vi "FuncImg-Export full data.vi"() -> (0 "error out":errorcluster, 11 "Exported file path":path)   [LabVIEW 2017]
uses:
  <userlib>/_MGI/File/MGI Windows Folder Enum.ctl
  Experiment header interface/Typedefs/Header parameters cluster-Zstack.ctl
  Typedefs/Frame Size.ctl
  Global variables/gl_Functional Imaging-Global variables.vi
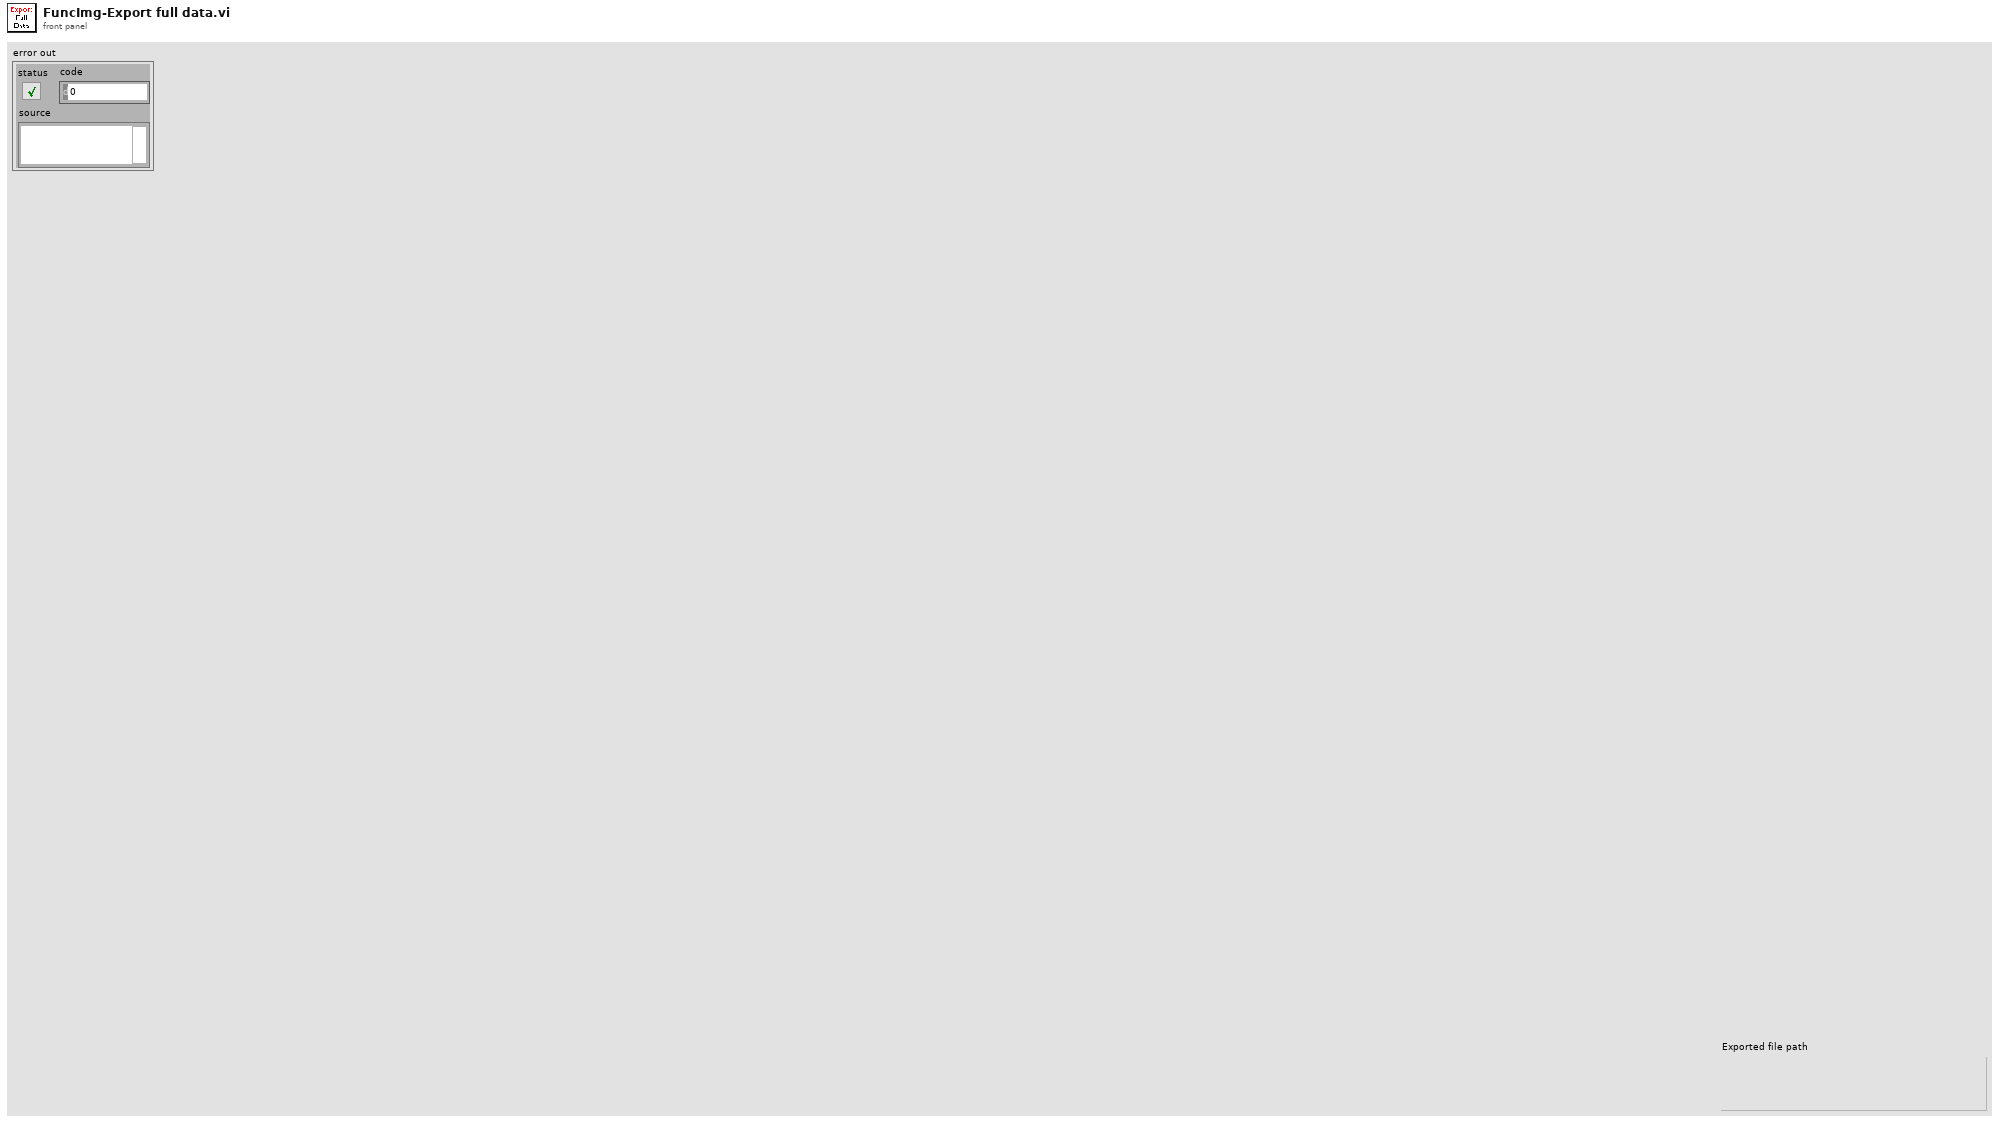
[diagram p1: front panel]
types:
  T1 = typedef "MGI Windows Folder Enum.ctl" = enum32{"Desktop", "Err<Internet>", "Programs", "Err<Controls>", "Err<Printers>", "Personal (MyDocuments)", "Favorites", "Startup", "Recent", "SendTo", "Err<RecycleBin>", "StartMenu", "Err<MyDocuments>", "MyMusic", "MyVideo", "Err<0x000F>", "DesktopDirectory", "Err<Drives>", "Err<Network>", "NetHood", "Fonts", "Templates", "CommonStartMenu", "CommonPrograms", "CommonStartup", "CommonDesktopDirectory", "AppData", "PrintHood", "LocalAppData", "Err<AltStartup>", "Err<CommonAltStartup>", "CommonFavorites", "InternetCache", "Cookies", "History", "CommonAppData", "Windows", "System", "ProgramFiles", "MyPictures", "Profile", "System32", "Err<0x002A>", "ProgramFilesCommon", "Err<0x002C>", "CommonTemplates", "CommonDocuments", "CommonAdminTools", "AdminTools"}
  T2 = typedef "Header parameters cluster-Zstack.ctl" = cluster{"Number of POI":u16, "Number of Miniscans":u16, "Number of Trials":u16, "Number of Cycles ":u16, "# Averaged Frames":u16, "Laser power (%)":u8, "Pockels":dbl, "Acquisition Length (sec)":dbl, "Fill time (us)":dbl, "DwellTime (us)":dbl, "Miniscan Dwell time per pixel (us)":dbl, "PMT 1":dbl, "PMT 2":dbl, "Back Apperture":dbl, "Zoom":dbl, "Number of Pixels in Miniscan":u16, "Frame Size":T3, "Field of View":dbl, "X centre":dbl, "Y centre":dbl, "AOL Z":dbl}
  T3 = typedef "Frame Size.ctl" = u16
  T4 = cluster{"Channel A?":bool, "Cycle length (us)":dbl, "[Pixels in ROI]":i32[], "Z-Stack Header data":T2, "[ROI Time (us)]":dbl[], "Path out":path, "Version index":i32}
  T5 = enum16{"open", "open or create", "create or replace", "create", "open (read-only)"}
  T6 = typedef "Functional Imging UI Refs.ctl" = cluster{"Menu ref":refnum<k9>, "Image control":refnum<vi>, "VI ref":refnum<vi>, "XGrapher":refnum<vi>, "Smoothing":refnum<vi>, "POI Averaging":refnum<vi>, "Normalize":refnum<vi>, "POI data points in each trial":refnum<vi>, "Channel":refnum<vi>, "Experiment data folder path":refnum<vi>, "[ROI vis]":refnum<vi>, "[Groups] visbl":T7, "Group Name":refnum<vi>, "POI index":refnum<vi>, "Trial No.":refnum<vi>, "Intensity Zoom":refnum<vi>, "Trial Cursor Enabled":refnum<vi>, "Number of Trials (ind 1)":refnum<vi>, "Number of Trials (ind 2)":refnum<vi>, "MiniScans Available":refnum<vi>, "POI Available":refnum<vi>, "Defer graph updates":refnum<vi>, "Waveform selector":refnum<vi>, "#of selected POI":refnum<vi>, "#of selected MiniScans":refnum<vi>, "#of selected groups":refnum<vi>, "Max Z-Projection":refnum<vi>, "Z-Plane Selector":refnum<vi>, "Index of miniscan point to visualise":refnum<vi>, "ROI vis. mode":refnum<vi>, "Total # of points":refnum<vi>, "Index of group clicked on":refnum<vi>, "Pane 1":refnum<vi>, "Pane 2":refnum<vi>, "Pane 3":refnum<vi>, "Pane 4":refnum<vi>, "Pane 5":refnum<vi>, "Pane 6":refnum<vi>, "Deselect all ROI":refnum<vi>, "Deselect all groups":refnum<vi>}
  T7 = typedef "Groups array referecne.ctl" = refnum<vi>
  T8 = typedef "ROI selector array-ROI vis.ctl" = T9[]
  T9 = typedef "Interface-ROI selection cluster.ctl" = cluster{"ROI number":i32, "ROI ID":T10, "Visibility":bool}
  T10 = typedef "ROI ID Enum.ctl" = enum16{"Point", "MiniScan", "Comp. MiniScan", "Rectangle", "Comp. volume", "Arb. plane point", "None"}
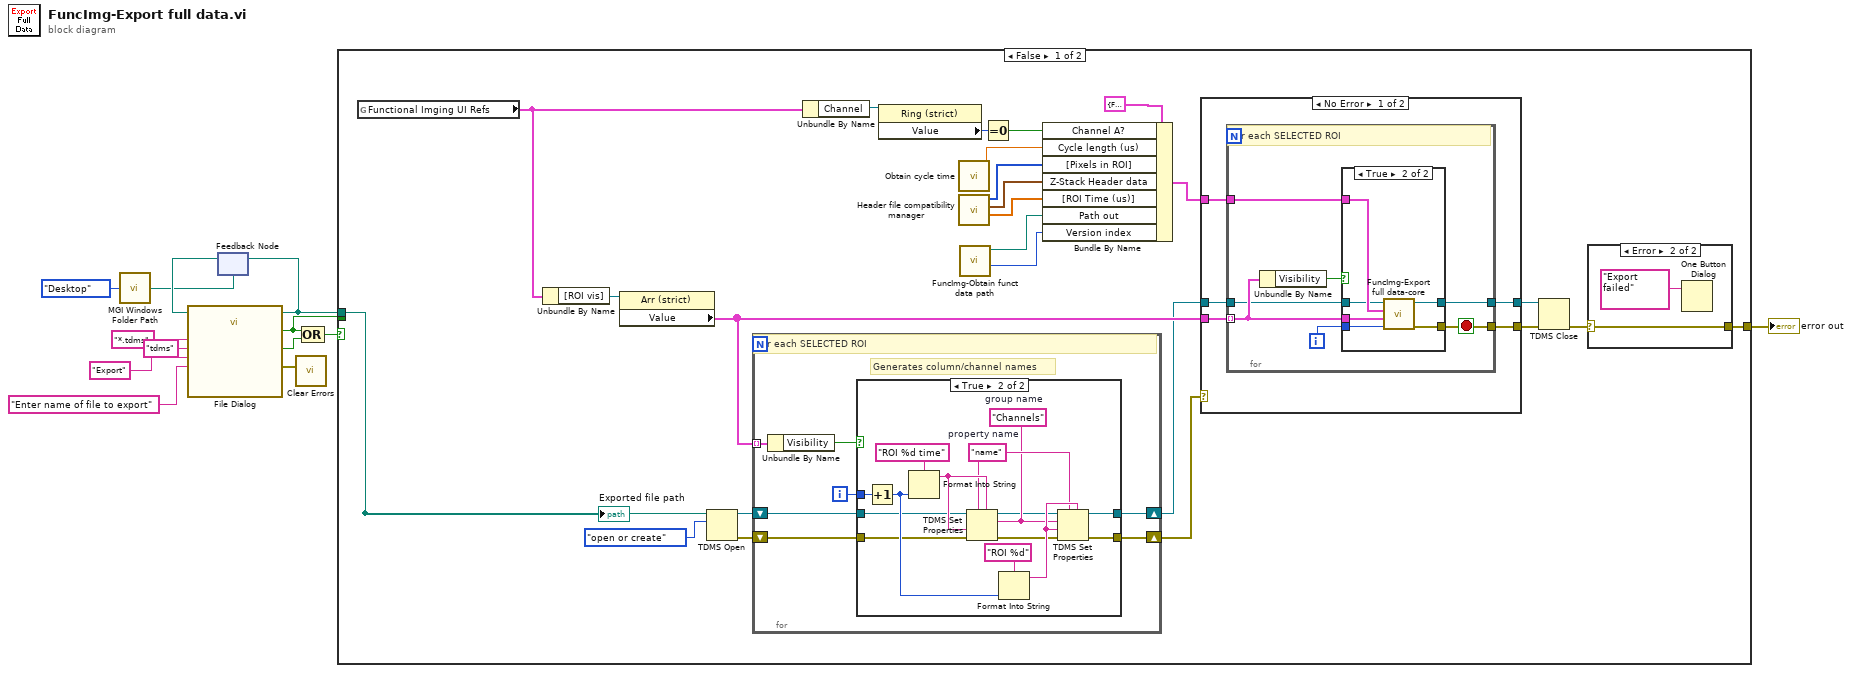
[diagram p0: block diagram]
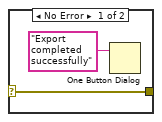
[diagram p2: hidden frame]
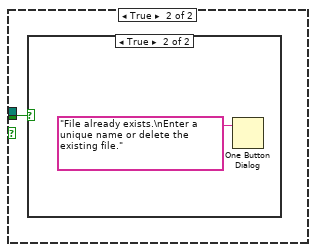
[diagram p6: hidden frame]
diagram:
  n1 = call <userlib>:"MGI Windows Folder Path.vi"("Windows Folder"=MGI_Windows_Folder_Enum."Desktop") -> ("Path"=w10:path)
  n2 = feedback #1(w10) -> (w12:path)
  n3 = call "File Dialog"("start path"=w12, "prompt"="Enter name of file to export", "button label"="Export", "pattern (all files)"="*.tdms" ("pattern label"), "pattern label"="tdms") -> ("selected path"=w1:path, "exists"=w2:bool, "cancelled"=w7:bool, "error out"=w8:errorcluster)  [unwired: 7 in]
  n4 = feedback-in #1(w1) -> ()
  n5 = call <vilib>:"Clear Errors.vi"("error in (no error)"=w8) -> ()  [unwired: 5 in, 2 out]
  n6 = Compound Arithmetic op=OR(w2, w7) -> (w6:bool)
  n7 = case shown="False" w6 {
    tunnel: [w15 _] -> w13
    tunnel: w2 -> [_ w86]
    tunnel: w1 -> [w17 _]
    frame False {
      n8 = global read "gl_Functional Imaging-Global variables.vi" "Functional Imging UI Refs"() -> (w30:T6)
      n9 = Unbundle By Name(w30) -> ("[ROI vis]"=w29:refnum<vi>)
      n10 = property on="Property Node" class="Arr (strict)"(reference=w29) -> ("Value"=w24:T8)  [unwired: 1 in, 2 out]
      n11 = TDMS Open(10:T5."open or create" ("operation (0:open)"), 11:w17) -> (0:w20:errorcluster, 3:w21:refnum<k34>)  [unwired: 5 in]
      n12 = for {
        tunnel: w24 -> [w69] mode=indexing
        shift-right: [w65] -> w19
        shift-left: w20 -> [w64]
        shift-right: [w63] -> w18
        shift-left: w21 -> [w66]
        i -> [w67]
        # "Generates column/channel names"
        # "For each SELECTED ROI"
        n13 = Unbundle By Name(w69) -> ("Visibility"=w68:bool)
        n14 = case shown="True" w68 {
          tunnel: w67 -> [_ w85]
          tunnel: w64 -> [w70 w76]
          tunnel: w66 -> [w71 w77]
          tunnel: [w71 w73] -> w63
          tunnel: [w70 w72] -> w65
          frame False {
          }
          frame True {
            w78 = "Channels"  # group name
            w79 = "name"  # property name
            n15 = Increment(x=w85) -> (x+1=w81:i32)
            n16 = Format Into String(format string="ROI %d time", w81) -> (resulting string=w80:string)  [unwired: 2 in, 1 out]
            n17 = TDMS Set Properties(5:w80, 7:w79, 8:w76, 9:w80, 10:w78, 11:w77) -> (0:w74:errorcluster, 3:w75:refnum<k34>)  [unwired: 2 out]
            n18 = Format Into String(format string="ROI %d", w81) -> (resulting string=w83:string)  [unwired: 2 in, 1 out]
            n19 = TDMS Set Properties(5:w83, 7:w79, 8:w74, 9:w83, 10:w78, 11:w75) -> (0:w72:errorcluster, 3:w73:refnum<k34>)  [unwired: 2 out]
          }
        }
      }
      n20 = Unbundle By Name(w30) -> ("Channel"=w28:refnum<vi>)
      n21 = property on="Property Node" class="Ring (strict)"(reference=w28) -> ("Value"=w36:u16)  [unwired: 1 in, 2 out]
      n22 = call "Obtain cycle time.vi"() -> ("Funct Acq cycle length (us)"=w31:dbl)  [unwired: 9 in, 2 out]
      n23 = call "Header file compatibility manager.vi"() -> ("[ROI Time (us)]"=w33:dbl[], "Z-Stack Header data"=w32:T2, "[Pixels in ROI]"=w27:i32[])  [unwired: 8 in, 1 out]
      n24 = call "FuncImg-Obtain funct data path.vi"() -> ("Version index (-1 = latest version)"=w35:i32, "Functional data folder path"=w34:path)  [unwired: 7 in, 3 out]
      n25 = Equal To 0?(x=w36) -> (x = 0?=w37:bool)
      n26 = Bundle By Name(cluster=T4 {"Channel A?"=FALSE, "Cycle length (us)"=0.0, "[Pixels in ROI]"=[], "Z-Stack Header data"={"Number of POI"=0, "Number of Miniscans"=0, "Number of Trials"=0, "Number of Cycles "=0, "# Averaged Frames"=0, "Laser power (%)"=0, "Pockels"=0.0, "Acquisition Length (sec)"=0.0, "Fill time (us)"=0.0, "DwellTime (us)"=0.0, "Miniscan Dwell time per pixel (us)"=0.0, "PMT 1"=0.0, "PMT 2"=0.0, "Back Apperture"=0.0, "Zoom"=0.0, "Number of Pixels in Miniscan"=0, "Frame Size"=200, "Field of View"=0.0, "X centre"=0.0, "Y centre"=0.0, "AOL Z"=0.0}, "[ROI Time (us)]"=[], "Path out"=path "", "Version index"=0} ("Cluster"), "Channel A?"=w37, "Cycle length (us)"=w31, "[Pixels in ROI]"=w27, "Z-Stack Header data"=w32, "[ROI Time (us)]"=w33, "Path out"=w34, "Version index"=w35) -> (w26:T4)
      n27 = case shown="No Error" w19 {
        selector: w19 -> [_ w62]
        tunnel: [w46 w62] -> w22
        tunnel: w26 -> [w45 _]
        tunnel: w24 -> [w44 _]
        tunnel: w18 -> [w43 w61]
        tunnel: [w42 w61] -> w23
        frame No Error {
          n28 = for {
            tunnel: w44 -> [w51] mode=indexing
            tunnel: w45 -> [w53]
            tunnel: [w52] -> w46
            tunnel: w43 -> [w49]
            tunnel: [w47] -> w42
            i -> [w48]
            stop <- w52 stop-if-true
            # "For each SELECTED ROI"
            n29 = Unbundle By Name(w51) -> ("Visibility"=w50:bool)
            n30 = case shown="True" w50 {
              tunnel: w51 -> [_ w58]
              tunnel: w53 -> [_ w60]
              tunnel: [_ w59] -> w52
              tunnel: w49 -> [w54 w57]
              tunnel: w48 -> [_ w56]
              tunnel: [w54 w55] -> w47
              frame False {
              }
              frame True {
                n31 = call "FuncImg-Export full data-core.vi"("FOR loop index"=w56, "System Cluster"=w58, "Input cluster"=w60, "Exported tdms file"=w57) -> ("error out"=w59:errorcluster, "Exported tdms file"=w55:refnum<k34>)  [unwired: 6 in]
              }
            }
          }
        }
        frame Error {
        }
      }
      n32 = TDMS Close(8:w22, 11:w23) -> (0:w16:errorcluster)  [unwired: 1 out]
      n33 = case shown="Error" w16 {
        selector: w16 -> [w39 w41]
        tunnel: [w39 w41] -> w15
        frame No Error {
          n34 = One Button Dialog(message="Export completed successfully") -> ()  [unwired: 1 in, 1 out]
        }
        frame Error {
          n35 = One Button Dialog(message="Export failed") -> ()  [unwired: 1 in, 1 out]
        }
      }
      "Exported file path" <- w17
    }
    frame True {
      n36 = case shown="True" w86 {
        frame False {
        }
        frame True {
          n37 = One Button Dialog(message="File already exists.\nEnter a unique name or delete the existing file.") -> ()  [unwired: 1 in, 1 out]
        }
      }
    }
  }
  "error out" <- w13
